vi "NI VeriStand - Get Channel Value by Data Reference.vi"(8 "error in (no error)":errorcluster, 11 "Data Reference in":T1 format="%.0x") -> (0 "error out":errorcluster, 2 "Value":dbl)   [LabVIEW 2020, in "Custom Device API.lvlib"]
doc: "Returns the value of the custom device channel specified by <B>Data Reference in</B>. Use the Get Channel Data Reference VI to get the channel data reference for this VI.\n\nYou can use this VI in the Execute Model case of an Inline Model Interface custom device, or in the Read Data from HW or Write Data to HW cases of an Inline Hardware Interface custom device. Do not use this VI outside of an inline custom device."
uses:
  <vilib>/NI VeriStand/Custom Device API/Custom Device API.lvlib
  <vilib>/NI VeriStand/Custom Device API/Data Reference.ctl
  <vilib>/NI VeriStand/Custom Device API/Global Data Refs.vi
  <vilib>/NI VeriStand/Custom Device API/data/NIVeriStand_DataServices.dll
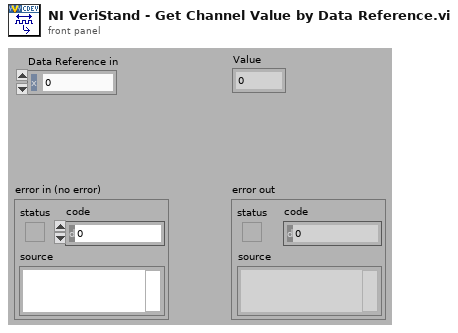
[diagram p1: front panel]
types:
  T1 = typedef "Custom Device API.lvlib/Data Reference.ctl" = i32
  T2 = typedef "Custom Device API.lvlib/Data Table Ref.ctl" = cluster{"Ptr.Beg":u64, "Ptr.End":u64}
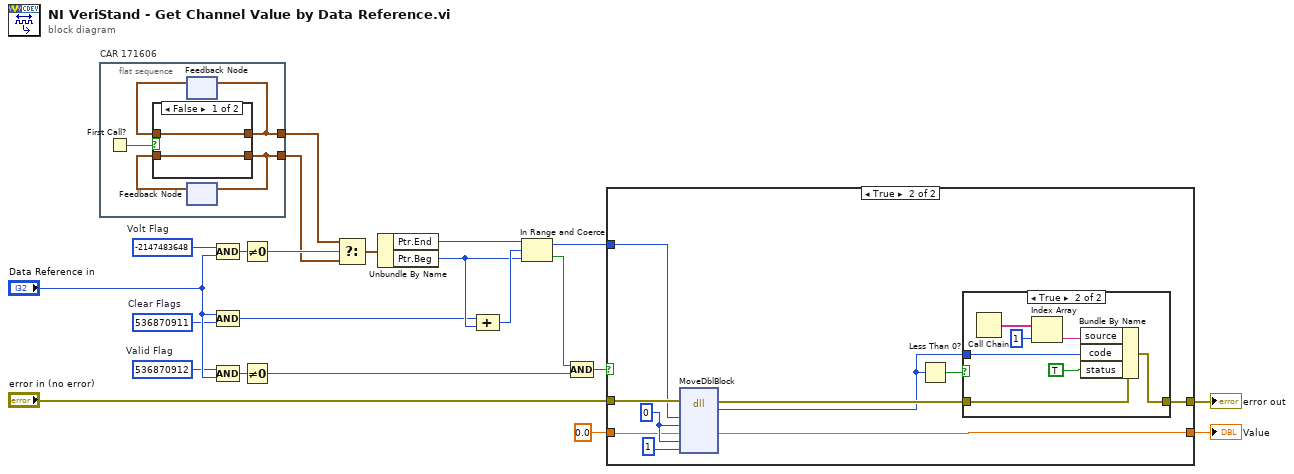
[diagram p0: block diagram]
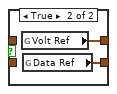
[diagram p2: hidden frame]
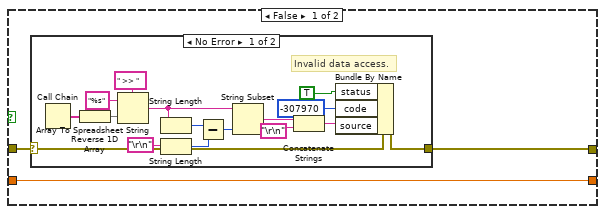
[diagram p3: hidden frame]
diagram:
  w3 = T1 536870912  # Valid Flag
  w4 = T1 536870911  # Clear Flags
  w5 = T1 -2147483648  # Volt Flag
  n1 = flat-sequence "CAR 171606" {
    tunnel: [w24] -> w2
    tunnel: [w23] -> w1
    frame #0 {
      n2 = First Call?() -> (First Call?: T/F=w27:bool)
      n3 = feedback #1() -> (w26:T2)  [unwired: 1 out]
      n4 = feedback #2() -> (w25:T2)  [unwired: 1 out]
      n5 = case shown="False" w27 {
        tunnel: [w29 w31] -> w24
        tunnel: w26 -> [w29 _]
        tunnel: [w28 w30] -> w23
        tunnel: w25 -> [w28 _]
        frame False {
        }
        frame True {
          n6 = global read "Global Data Refs.vi" "Volt Ref"() -> (w31:T2)
          n7 = global read "Global Data Refs.vi" "Data Ref"() -> (w30:T2)
        }
      }
      n8 = feedback-in #1(w24) -> ()
      n9 = feedback-in #2(w23) -> ()
    }
  }
  n10 = Compound Arithmetic op=AND(w5, "Data Reference in") -> (w12:T1)
  n11 = Compound Arithmetic op=AND("Data Reference in", w4) -> (w6:T1)
  n12 = Compound Arithmetic op=AND(w3, "Data Reference in") -> (w8:T1)
  n13 = Not Equal To 0?(x=w12) -> (x != 0?=w11:bool)
  n14 = Not Equal To 0?(x=w8) -> (x != 0?=w7:bool)
  n15 = Select(t=w2, s=w11, f=w1) -> (s? t:f=w10:T2)
  n16 = Unbundle By Name(w10) -> ("Ptr.End"=w14:u64, "Ptr.Beg"=w13:u64)
  n17 = Compound Arithmetic op=ADD(w6, w13) -> (w17:u64)
  n18 = In Range and Coerce(upper limit=w14, x=w17, lower limit=w13) -> (coerced(x)=w16:u64, In Range?=w15:bool)
  n19 = Compound Arithmetic op=AND(w15, w7) -> (w9:bool)
  n20 = case shown="True" w9 {
    tunnel: "error in (no error)" -> [w32 w61]
    tunnel: [w33 w53] -> w22
    tunnel: [w34 w56] -> w19
    tunnel: w16 -> [_ w60]
    tunnel: 0.0 ("pd") -> [w34 w57]
    frame False {
      n21 = case shown="No Error" w32 {
        selector: w32 -> [w47 w51]
        tunnel: [w50 w51] -> w33
        frame No Error {
          # "Invalid data access."
          n22 = Call Chain() -> (call chain=w36:string[])
          n23 = Reverse 1D Array(array=w36) -> (reversed array=w43:string[])
          n24 = Array To Spreadsheet String(delimiter (Tab)=" >> ", array=w43, 3:"%s" ("format string")) -> (spreadsheet string=w44:string)
          n25 = String Length(string=w44) -> (length=w42:i32)
          n26 = String Length(string="\r\n") -> (length=w46:i32)
          n27 = Subtract(x=w42, y=w46) -> (x-y=w41:i32)
          n28 = String Subset(string=w44, length (rest)=w41) -> (substring=w37:string)  [unwired: 1 out]
          n29 = Concatenate Strings(w37, "\r\n") -> (w35:string)
          n30 = Bundle By Name(cluster=w47, "status"=TRUE, "code"=-307970, "source"=w35) -> (w50:errorcluster)
        }
        frame Error {
          # "Leave existing error."
        }
      }
    }
    frame True {
      w58 = u64 0 ("size")
      n31 = dll-call lib="e:/penguin/lvtoolchain/2020/eng32/export/20.0/20.0.0f11/win/vi.lib/NI VeriStand/Custom Device API/data/NIVeriStand_DataServices.*" fn="MoveDblBlock"(error in=w61, "srcPtr"=w60, "srcOffset"=w58, "dstPtr"=w57, "dstOffset"=w58, "count"=u64 1 ("size")) -> (error out=w54:errorcluster, "return type"=w52:i32, "dstPtr"=w56:dbl)  [unwired: 6 in, 1 out]
      n32 = Less Than 0?(x=w52) -> (x < 0?=w55:bool)
      n33 = case shown="True" w55 {
        tunnel: w54 -> [w62 w67]
        tunnel: w52 -> [_ w64]
        tunnel: [w62 w66] -> w53
        frame False {
        }
        frame True {
          n34 = Call Chain() -> (call chain=w68:string[])
          n35 = Index Array(array=w68, index=1) -> (element=w63:string)
          n36 = Bundle By Name(cluster=w67, "source"=w63, "code"=w64, "status"=TRUE) -> (w66:errorcluster)
        }
      }
    }
  }
  "Value" <- w19
  "error out" <- w22
